vi "Handle Event.vi"(8 "error in":errorcluster, 9 "data":variant, 10 "event":variant, 11 "module reference in":T1) -> (0 "error out":errorcluster, 3 "module reference out":T1)   [LabVIEW 2017, in "Controller.lvlib"]
uses:
  Controller.lvlib
  Private TypeDefs/Module Reference.ctl
  Global TypeDefs/Registered Modules.ctl
  Private TypeDefs/Module Queues.ctl
  Private TypeDefs/Message Queue Element.ctl
  Private TypeDefs/Messages.ctl
  Private TypeDefs/Module Notifiers.ctl
  Private TypeDefs/Dummy Notifier.ctl
  Private TypeDefs/Event and Data.ctl
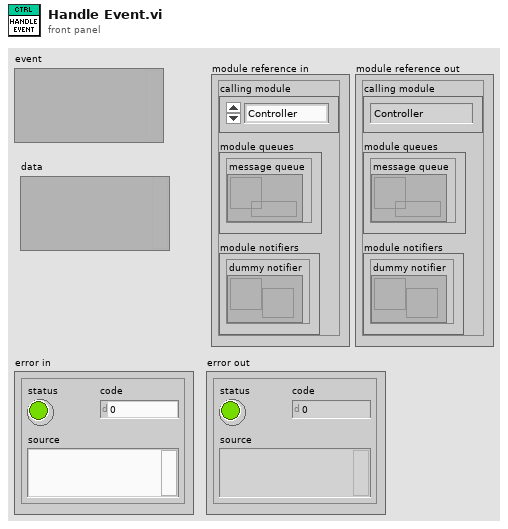
[diagram p1: front panel]
types:
  T1 = typedef "Controller.lvlib/Module Reference.ctl" = cluster{"calling module":T2, "module queues":T3, "module notifiers":T4}
  T2 = typedef "Registered Modules.ctl" = enum16{"Controller", "DAQ", "Error Handler", "Game", "myPAM", "WinHost", "Logger"}
  T3 = typedef "Controller.lvlib/Module Queues.ctl" = cluster{"message queue":refnum<queue>}
  T4 = typedef "Controller.lvlib/Module Notifiers.ctl" = cluster{"dummy notifier":refnum<notifier>}
  T5 = typedef "Controller.lvlib/Messages.ctl" = enum16{"shutdown", "handle event", "start system"}
  T6 = typedef "Controller.lvlib/Event and Data.ctl" = cluster{"event":variant, "data":variant}
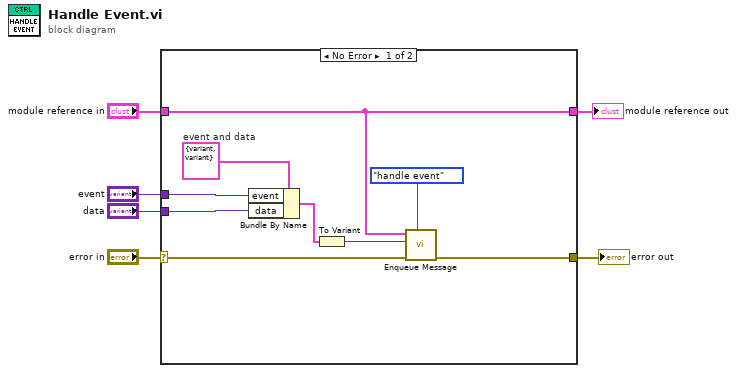
[diagram p0: block diagram]
diagram:
  n1 = case shown="No Error" "error in" {
    selector: "error in" -> [w15 w17]
    tunnel: [w7 w17] -> w1
    tunnel: "module reference in" -> [w13 w16]
    tunnel: [w13 w16] -> w4
    tunnel: "event" -> [w11 _]
    tunnel: "data" -> [w10 _]
    frame No Error {
      w12 = T6 {"event"=variant, "data"=variant}  # event and data
      n2 = Bundle By Name(cluster=w12, "event"=w11, "data"=w10) -> (w9:T6)
      n3 = To Variant(anything=w9) -> (Variant=w8:variant)
      n4 = call "Enqueue Message.vi"("message"=Messages."handle event", "error in"=w15, "data"=w8, "module reference in"=w13) -> ("error out"=w7:errorcluster)  [unwired: 6 in, 1 out]
    }
    frame Error {
    }
  }
  "module reference out" <- w4
  "error out" <- w1
